vi "Read State Machine Status.vi"(8 "error in (no error)":errorcluster, 11 "Command State in":refnum<class "State Machine.lvclass">) -> (0 "error out":errorcluster, 2 "State Machine Status":T1, 3 "Command State out":refnum<class "State Machine.lvclass">)   [LabVIEW 2013, in "State Machine.lvclass"]
uses:
  State Machine.lvclass
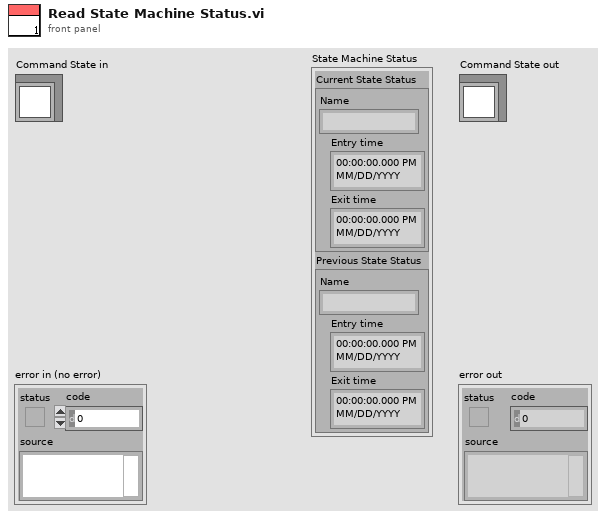
[diagram p1: front panel]
types:
  T1 = cluster{"Current State Status":cluster{"Name":string, "Entry time":timestamp, "Exit time":timestamp}, "Previous State Status":cluster{"Name":string, "Entry time":timestamp, "Exit time":timestamp}}
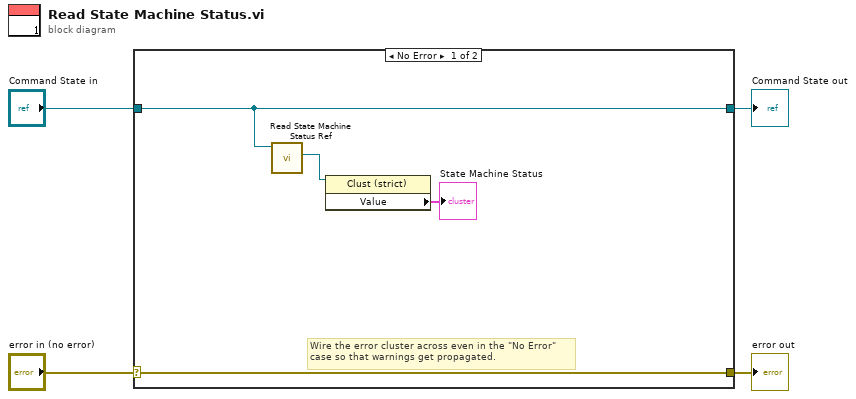
[diagram p0: block diagram]
diagram:
  n1 = case shown="No Error" "error in (no error)" {
    selector: "error in (no error)" -> [w8 w10]
    tunnel: [w8 w10] -> w3
    tunnel: [w7 w9] -> w1
    tunnel: "Command State in" -> [w7 w9]
    frame No Error {
      # "Wire the error cluster across even in the \"No Error\"\ncase so that warnings get propagated."
      n2 = call-dynamic "Read State Machine Status Ref.vi"("State Machine in"=w7) -> ("State Machine Status Ref"=w6:refnum<vi>)  [unwired: 8 in, 2 out]
      n3 = property class="Clust (strict)"(reference=w6) -> ("Value"=→"State Machine Status":T1)  [unwired: 1 in, 2 out]
    }
    frame Error {
    }
  }
  "error out" <- w3
  "Command State out" <- w1
